vi "Pot Line.vi"(7 "Encapsulant":string, 8 "error in (no error)":errorcluster, 9 "End Position":refnum<class "Vec3d.lvclass">, 10 "Start Position":refnum<class "Vec3d.lvclass">, 11 "Gantry in":refnum<class "Gantry.lvclass">) -> (0 "error out":errorcluster, 3 "Gantry out":refnum<class "Gantry.lvclass">)   [LabVIEW 2024, in "Gantry.lvclass"]
uses:
  Gantry.lvclass
  Vec3d Class/Vec3d.lvclass
  FlexWorktable/FlexWorktable.lvclass
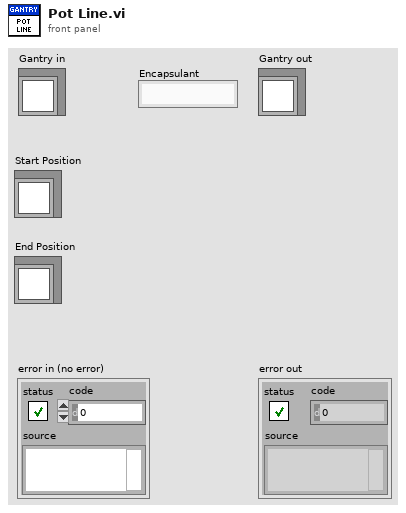
[diagram p1: front panel]
types:
  T1 = cluster{"Syringe Holder":string, "Mixing Time":timestamp, "Tip Offset":refnum<class "Vec3d.lvclass">}
  T2 = typedef "FlexWorktable.lvclass/Potting Parameters.ctl" = cluster{"Curing Param A":dbl, "Curing Param B":dbl, "Speed Nominal":dbl, "Time Nominal":dbl, "Turn-on Time":dbl, "Turn-off Time":dbl, "Safe Height Offset":dbl, "Tip Height":dbl}
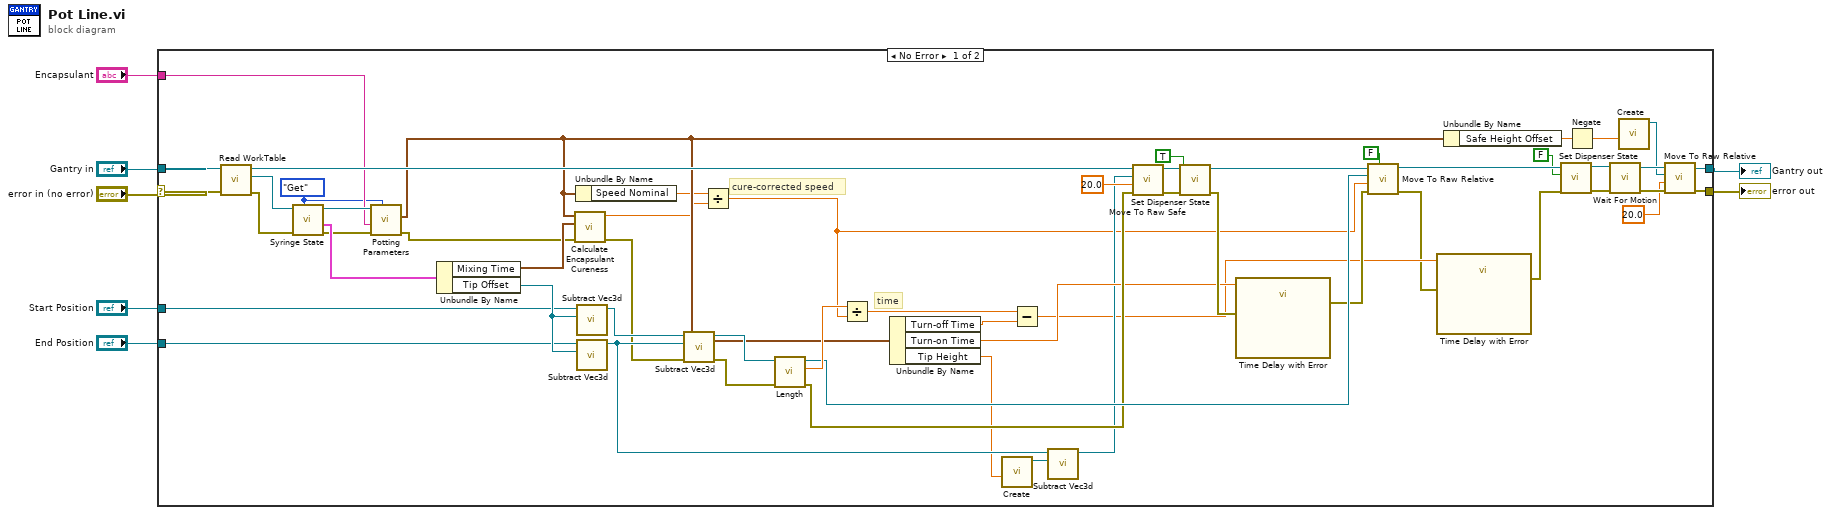
[diagram p0: block diagram]
diagram:
  n1 = case shown="No Error" "error in (no error)" {
    selector: "error in (no error)" -> [w20 w65]
    tunnel: [w53 w65] -> w1
    tunnel: [w57 w64] -> w2
    tunnel: "Gantry in" -> [w21 w64]
    tunnel: "End Position" -> [w28 _]
    tunnel: "Start Position" -> [w27 _]
    tunnel: "Encapsulant" -> [w19 _]
    frame No Error {
      w17 = enum16{"Get", "Set"}."Get" ("Get/Set")
      # "cure-corrected speed"
      # "time"
      n2 = call-dynamic "Read WorkTable.vi"("error in"=w20, "Gantry Class in"=w21) -> ("error out"=w24:errorcluster, "Worktable"=w25:refnum<class "FlexWorktable.lvclass">, "Gantry Class out"=w51:refnum<class "Gantry.lvclass">)  [unwired: 7 in]
      n3 = call-dynamic "Syringe State.vi"("Get/Set"=w17, "error in (no error)"=w24, "FlexWorktable in"=w25) -> ("error out"=w18:errorcluster, "Syringe out"=w23:T1, "FlexWorktable out"=w22:refnum<class "FlexWorktable.lvclass">)  [unwired: 6 in]
      n4 = call-dynamic "Potting Parameters.vi"("Get/Set"=w17, "error in (no error)"=w18, "Encapsulant"=w19, "FlexWorktable in"=w22) -> ("error out"=w15:errorcluster, "Potting Parameters out"=w13:T2)  [unwired: 5 in, 1 out]
      n5 = Unbundle By Name(w23) -> ("Mixing Time"=w16:timestamp, "Tip Offset"=w50:refnum<class "Vec3d.lvclass">)
      n6 = call "Calculate Encapsulant Cureness.vi"("error in"=w15, "Mixing Time"=w16, "Potting Parameters"=w13) -> ("error out"=w14:errorcluster, "Cureness"=w11:dbl)  [unwired: 7 in]
      n7 = Unbundle By Name(w13) -> ("Speed Nominal"=w12:dbl)
      n8 = call "Subtract Vec3d.vi"("Vec3d in 2"=w50, "Vec3d in 1"=w27) -> ("Vec3d Class out"=w52:refnum<class "Vec3d.lvclass">)  [unwired: 8 in, 1 out]
      n9 = call "Subtract Vec3d.vi"("Vec3d in 2"=w50, "Vec3d in 1"=w28) -> ("Vec3d Class out"=w35:refnum<class "Vec3d.lvclass">)  [unwired: 8 in, 1 out]
      n10 = call "Subtract Vec3d.vi"("error in (no error)"=w14, "Vec3d in 2"=w35, "Vec3d in 1"=w52) -> ("error out"=w49:errorcluster, "Vec3d Class out"=w62:refnum<class "Vec3d.lvclass">)  [unwired: 7 in]
      n11 = Divide(x=w12, y=w11) -> (x/y=w10:dbl)
      n12 = call-dynamic "Length.vi"("error in"=w49, "Vec3d in"=w62) -> ("error out"=w48:errorcluster, "Length"=w63:dbl, "Vec3d out"=w61:refnum<class "Vec3d.lvclass">)  [unwired: 7 in]
      n13 = Divide(x=w63, y=w10) -> (x/y=w60:dbl)
      n14 = Unbundle By Name(w13) -> ("Turn-off Time"=w39:dbl, "Turn-on Time"=w38:dbl, "Tip Height"=w29:dbl)
      n15 = call "Create.vi"("Z"=w29) -> ("Vec3d Class out"=w33:refnum<class "Vec3d.lvclass">)  [unwired: 9 in, 1 out]
      n16 = Subtract(x=w60, y=w39) -> (x-y=w32:dbl)
      n17 = call "Subtract Vec3d.vi"("Vec3d in 2"=w33, "Vec3d in 1"=w35) -> ("Vec3d Class out"=w34:refnum<class "Vec3d.lvclass">)  [unwired: 8 in, 1 out]
      n18 = call-dynamic "Move To Raw Safe.vi"("error in"=w48, "Speed(mm/s)"=20.0, "Destination"=w34, "Gantry in"=w51) -> ("error out"=w46:errorcluster, "Gantry out"=w45:refnum<class "Gantry.lvclass">)  [unwired: 6 in]
      n19 = call-dynamic "Set Dispenser State.vi"("error in"=w46, "On/Off"=TRUE, "Gantry in"=w45) -> ("error out"=w47:errorcluster, "Gantry out"=w59:refnum<class "Gantry.lvclass">)  [unwired: 7 in]
      n20 = call "Time Delay with Error.vi"("error in (no error)"=w47, "Delay Time (s)"=w38) -> ("error out"=w55:errorcluster)  [unwired: 9 in]
      n21 = call-dynamic "Move To Raw Relative.vi"("Wait?"=FALSE, "error in"=w55, "Speed(mm/s)"=w10, "Delta"=w61, "Gantry in"=w59) -> ("error out"=w31:errorcluster, "Gantry out"=w58:refnum<class "Gantry.lvclass">)  [unwired: 5 in]
      n22 = call "Time Delay with Error.vi"("error in (no error)"=w31, "Delay Time (s)"=w32) -> ("error out"=w30:errorcluster)  [unwired: 9 in]
      n23 = Unbundle By Name(w13) -> ("Safe Height Offset"=w26:dbl)
      n24 = call-dynamic "Set Dispenser State.vi"("error in"=w30, "On/Off"=FALSE, "Gantry in"=w58) -> ("error out"=w43:errorcluster, "Gantry out"=w42:refnum<class "Gantry.lvclass">)  [unwired: 7 in]
      n25 = Negate(x=w26) -> (-x=w40:dbl)
      n26 = call-dynamic "Wait For Motion.vi"("error in"=w43, "Gantry in"=w42) -> ("error out"=w54:errorcluster, "Gantry out"=w56:refnum<class "Gantry.lvclass">)  [unwired: 8 in]
      n27 = call "Create.vi"("Z"=w40) -> ("Vec3d Class out"=w41:refnum<class "Vec3d.lvclass">)  [unwired: 9 in, 1 out]
      n28 = call-dynamic "Move To Raw Relative.vi"("error in"=w54, "Speed(mm/s)"=20.0, "Delta"=w41, "Gantry in"=w56) -> ("error out"=w53:errorcluster, "Gantry out"=w57:refnum<class "Gantry.lvclass">)  [unwired: 6 in]
    }
    frame Error {
    }
  }
  "error out" <- w1
  "Gantry out" <- w2
